vi "get_counter_settings.vi"(8 "error in (no error)":errorcluster, 11 "TrajectoryDL091126GenericVoxel in":refnum<class "TrajectoryDL091126GenericVoxel.lvclass">) -> (0 "error out":errorcluster, 2 "counter settings":T1[](array[typedef]), 3 "TrajectoryDL091126GenericVoxel out":refnum<class "TrajectoryDL091126GenericVoxel.lvclass">)   [LabVIEW 2010, in "TrajectoryDL091126GenericVoxel.lvclass"]
uses:
  TrajectoryDL091126GenericVoxel.lvclass
  common/clusters/counter_settings_cluster.ctl
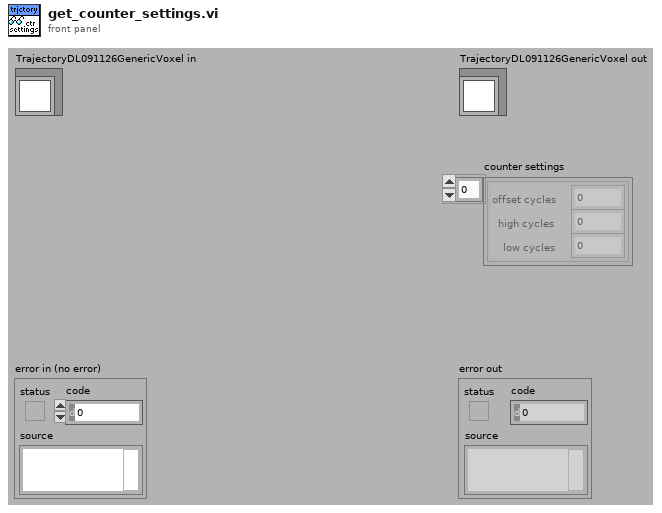
[diagram p1: front panel]
types:
  T1 = typedef "counter_settings_cluster.ctl" = cluster{"offset cycles":i32, "high cycles":i32, "low cycles":i32}
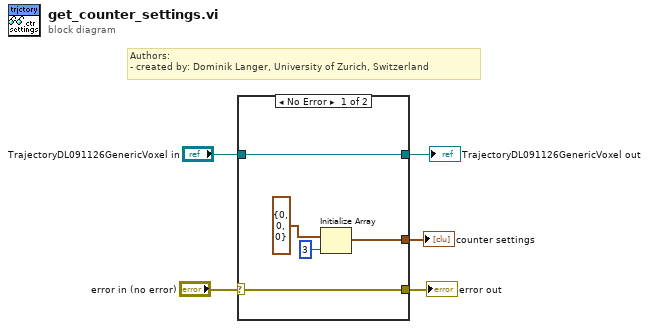
[diagram p0: block diagram]
diagram:
  # "Authors: \n- created by: Dominik Langer, University of Zurich, Switzerland"
  n1 = case shown="No Error" "error in (no error)" {
    selector: "error in (no error)" -> [w9 w12]
    tunnel: [w9 w12] -> w4
    tunnel: [w10 w11] -> w2
    tunnel: "TrajectoryDL091126GenericVoxel in" -> [w10 w11]
    tunnel: [w8 _] -> w1
    frame No Error {
      n2 = Initialize Array(T1 {"offset cycles"=0, "high cycles"=0, "low cycles"=0} ("counter"), 3 ("dimension size")) -> (w8:T1[])
    }
    frame Error {
    }
  }
  "error out" <- w4
  "TrajectoryDL091126GenericVoxel out" <- w2
  "counter settings" <- w1
